vi "WAIT_HOT.vi"(10 "argv":string[](array[string]), 11 "args":u8) -> ()   [LabVIEW 2014]
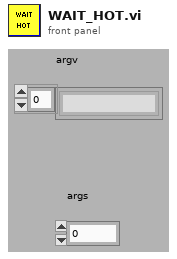
[diagram p1: front panel]
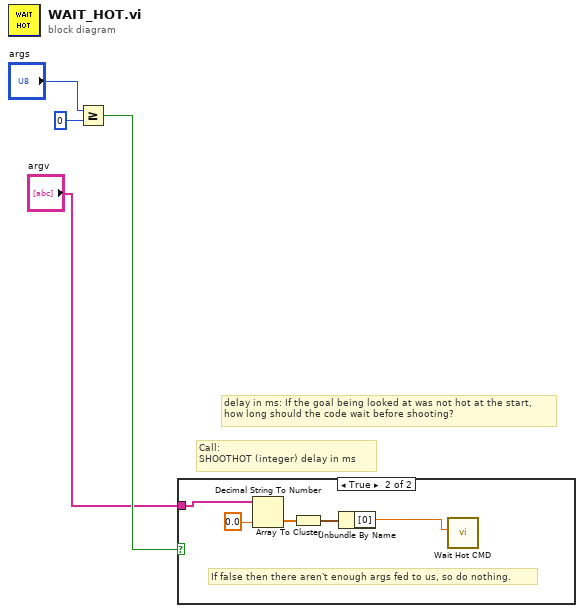
[diagram p0: block diagram]
diagram:
  # "delay in ms: If the goal being looked at was not hot at the start,\nhow long should the code wait before shooting?"
  # "Call:\nSHOOTHOT (integer) delay in ms"
  n1 = Greater Or Equal?(x="args", y=u8 0) -> (x >= y?=w4:bool)
  n2 = case shown="True" w4 {
    tunnel: "argv" -> [_ w6]
    frame False {
    }
    frame True {
      # "If false then there aren't enough args fed to us, so do nothing."
      n3 = Decimal String To Number(string=w6, default (0L)=0.0 ("default (0 I32)")) -> (number=w8:dbl[])  [unwired: 2 out]
      n4 = Array To Cluster(array=w8) -> (cluster=w7:cluster{"[0]":dbl, "[1]":dbl})
      n5 = Unbundle By Name(w7) -> ("[0]"=w5:dbl)
      n6 = call "Wait Hot CMD.vi"("Delay ms"=w5) -> ()  [unwired: 11 in]
    }
  }
